vi "Hot.vi"(8 "error in (no error)":errorcluster) -> (0 "error out":errorcluster, 1 "R Hot":bool, 2 "L Hot":bool, 3 "Hot?":bool)   [LabVIEW 2013]
uses:
  VisionData.ctl
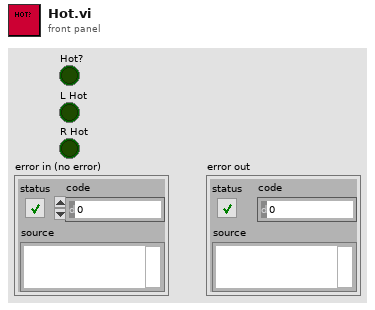
[diagram p1: front panel]
types:
  T1 = typedef "VisionData.ctl" = cluster{"Total":u8, "Timestamp":u32, "Horizontal":u8, "Vertical":u8, "Left Hot":bool, "Right Hot":bool}
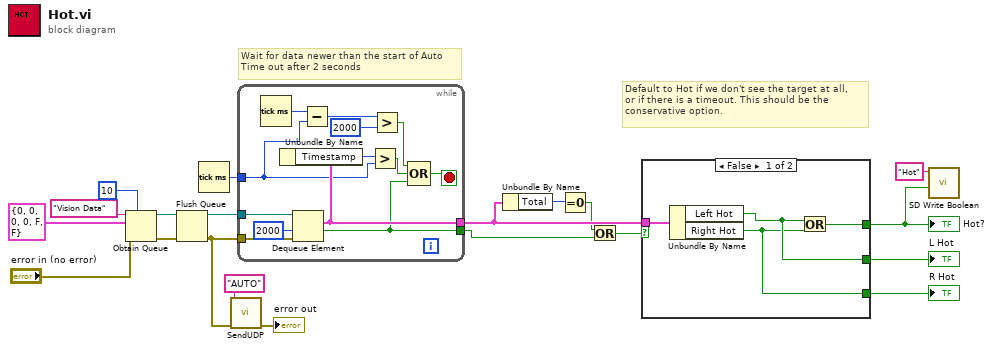
[diagram p0: block diagram]
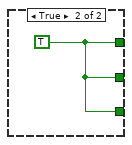
[diagram p2: hidden frame]
diagram:
  # "Wait for data newer than the start of Auto\nTime out after 2 seconds"
  # "Default to Hot if we don't see the target at all, \nor if there is a timeout. This should be the \nconservative option."
  n1 = Obtain Queue(max queue size (-1, unlimited)=10, name (unnamed)="Vision Data", element data type=T1 {"Total"=0, "Timestamp"=0, "Horizontal"=0, "Vertical"=0, "Left Hot"=FALSE, "Right Hot"=FALSE}, error in (no error)="error in (no error)") -> (queue out=w16:refnum<queue>, error out=w18:errorcluster)  [unwired: 1 in, 1 out]
  n2 = Flush Queue(queue=w16, error in (no error)=w18) -> (queue out=w17:refnum<queue>, error out=w19:errorcluster)  [unwired: 1 out]
  n3 = Tick Count (ms)() -> (millisecond timer value=w11:u32)
  n4 = call "SendUDP.vi"("error in (no error)"=w19, "data in"="AUTO") -> ("error out"=→"error out":errorcluster)  [unwired: 9 in]
  n5 = while {
    tunnel: [w27] -> w3
    tunnel: [w30] -> w7
    tunnel: w19 -> [w33]
    tunnel: w17 -> [w31]
    tunnel: w11 -> [w24]
    stop <- w26 stop-if-true
    n6 = Tick Count (ms)() -> (millisecond timer value=w25:u32)
    n7 = Dequeue Element(queue=w31, timeout in ms (-1)=2000, error in (no error)=w33) -> (element=w30:T1, timed out?=w27:bool)  [unwired: 2 out]
    n8 = Unbundle By Name(w30) -> ("Timestamp"=w29:u32)
    n9 = Subtract(x=w25, y=w24) -> (x-y=w23:u32)
    n10 = Greater?(x=w29, y=w24) -> (0:w28:bool)
    n11 = Greater?(x=w23, y=u32 2000) -> (0:w21:bool)
    n12 = Compound Arithmetic op=OR(w21, w28, w27) -> (w26:bool)
  }
  n13 = Unbundle By Name(w7) -> ("Total"=w6:u8)
  n14 = Equal To 0?(x=w6) -> (x = 0?=w4:bool)
  n15 = Or(x=w4, y=w3) -> (x .or. y?=w5:bool)
  n16 = case shown="False" w5 {
    tunnel: w7 -> [w37 _]
    tunnel: [w36 w38] -> w10
    tunnel: [w35 w38] -> w9
    tunnel: [w34 w38] -> w8
    frame False {
      n17 = Unbundle By Name(w37) -> ("Left Hot"=w35:bool, "Right Hot"=w34:bool)
      n18 = Or(x=w35, y=w34) -> (x .or. y?=w36:bool)
    }
    frame True {
      w38 = TRUE
    }
  }
  "Hot?" <- w10
  "R Hot" <- w8
  "L Hot" <- w9
  n19 = call <vilib>:"SD Write Boolean.vi"("Boolean"=w10, "Name"="Hot") -> ()  [unwired: 8 in, 2 out]
